vi "CAN MESSAGE.vi"(0 "interface":refnum<k21>, 1 "CAN frame":T1 {"payload" format="%x"; "timestamp" format="%<%.7X\n%x>T"; "type" items=["CAN Data"=0, "CAN Remote"=1, "CAN Bus Error"=2, "CAN 2.0 Data"=8, "CAN FD Data"=16, "CAN FD+BRS Data"=24, "J1939 Data"=192, "Delay"=224, "Log Trigger"=225, "Start Trigger"=226]; "identifier" format="%x"}) -> (2 "cluster":T3 {"data[0]"."payload" format="%x"; "data[0]"."timestamp" format="%<%.7X\n%x>T"; "data[0]"."type" items=["CAN Data"=0, "CAN Remote"=1, "CAN Bus Error"=2, "CAN 2.0 Data"=8, "CAN FD Data"=16, "CAN FD+BRS Data"=24, "J1939 Data"=192, "Delay"=224, "Log Trigger"=225, "Start Trigger"=226]; "data[0]"."identifier" format="%x"; "data[1]"."payload" format="%x"; "data[1]"."timestamp" format="%<%.7X\n%x>T"; "data[1]"."type" items=["CAN Data"=0, "CAN Remote"=1, "CAN Bus Error"=2, "CAN 2.0 Data"=8, "CAN FD Data"=16, "CAN FD+BRS Data"=24, "J1939 Data"=192, "Delay"=224, "Log Trigger"=225, "Start Trigger"=226]; "data[1]"."identifier" format="%x"; "data[2]"."payload" format="%x"; "data[2]"."timestamp" format="%<%.7X\n%x>T"; "data[2]"."type" items=["CAN Data"=0, "CAN Remote"=1, "CAN Bus Error"=2, "CAN 2.0 Data"=8, "CAN FD Data"=16, "CAN FD+BRS Data"=24, "J1939 Data"=192, "Delay"=224, "Log Trigger"=225, "Start Trigger"=226]; "data[2]"."identifier" format="%x"; "data[3]"."payload" format="%x"; "data[3]"."timestamp" format="%<%.7X\n%x>T"; "data[3]"."type" items=["CAN Data"=0, "CAN Remote"=1, "CAN Bus Error"=2, "CAN 2.0 Data"=8, "CAN FD Data"=16, "CAN FD+BRS Data"=24, "J1939 Data"=192, "Delay"=224, "Log Trigger"=225, "Start Trigger"=226]; "data[3]"."identifier" format="%x"; "data[4]"."payload" format="%x"; "data[4]"."timestamp" format="%<%.7X\n%x>T"; "data[4]"."type" items=["CAN Data"=0, "CAN Remote"=1, "CAN Bus Error"=2, "CAN 2.0 Data"=8, "CAN FD Data"=16, "CAN FD+BRS Data"=24, "J1939 Data"=192, "Delay"=224, "Log Trigger"=225, "Start Trigger"=226]; "data[4]"."identifier" format="%x"; "data[5]"."payload" format="%x"; "data[5]"."timestamp" format="%<%.7X\n%x>T"; "data[5]"."type" items=["CAN Data"=0, "CAN Remote"=1, "CAN Bus Error"=2, "CAN 2.0 Data"=8, "CAN FD Data"=16, "CAN FD+BRS Data"=24, "J1939 Data"=192, "Delay"=224, "Log Trigger"=225, "Start Trigger"=226]; "data[5]"."identifier" format="%x"; "data[6]"."payload" format="%x"; "data[6]"."timestamp" format="%<%.7X\n%x>T"; "data[6]"."type" items=["CAN Data"=0, "CAN Remote"=1, "CAN Bus Error"=2, "CAN 2.0 Data"=8, "CAN FD Data"=16, "CAN FD+BRS Data"=24, "J1939 Data"=192, "Delay"=224, "Log Trigger"=225, "Start Trigger"=226]; "data[6]"."identifier" format="%x"; "data[7]"."payload" format="%x"; "data[7]"."timestamp" format="%<%.7X\n%x>T"; "data[7]"."type" items=["CAN Data"=0, "CAN Remote"=1, "CAN Bus Error"=2, "CAN 2.0 Data"=8, "CAN FD Data"=16, "CAN FD+BRS Data"=24, "J1939 Data"=192, "Delay"=224, "Log Trigger"=225, "Start Trigger"=226]; "data[7]"."identifier" format="%x"; "data[8]"."payload" format="%x"; "data[8]"."timestamp" format="%<%.7X\n%x>T"; "data[8]"."type" items=["CAN Data"=0, "CAN Remote"=1, "CAN Bus Error"=2, "CAN 2.0 Data"=8, "CAN FD Data"=16, "CAN FD+BRS Data"=24, "J1939 Data"=192, "Delay"=224, "Log Trigger"=225, "Start Trigger"=226]; "data[8]"."identifier" format="%x"}, 4 "error out":errorcluster)   [LabVIEW 2022 SP3]
uses:
  <vilib>/xnet/xnet.llb/XNET Frame CAN.ctl
  <vilib>/xnet/xnet.llb/XNET Frame Type CAN.ctl
  <vilib>/xnet/xnet.llb/XNET Create Session (Frame Input Stream).vi
  <vilib>/xnet/xnet.llb/XNET Create Session (Frame Output Queued).vi
  <vilib>/xnet/xnet.llb/XNET Write (Frame CAN).vi
  <vilib>/xnet/xnet.llb/XNET Read (Frame CAN).vi
  <resource>/objmgr/xnet.rc
panel:
  in  "error in (no error) 2":errorcluster
  in  "error in (no error)":errorcluster
  in  "DATA IN":T1[](array[typedef]) {"payload" format="%x"; "timestamp" format="%<%.7X\n%x>T"; "type" items=["CAN Data"=0, "CAN Remote"=1, "CAN Bus Error"=2, "CAN 2.0 Data"=8, "CAN FD Data"=16, "CAN FD+BRS Data"=24, "J1939 Data"=192, "Delay"=224, "Log Trigger"=225, "Start Trigger"=226]; "identifier" format="%x"}
  out "data 2":T1[](array[typedef]) {"payload" format="%x"; "timestamp" format="%<%.7X\n%x>T"; "type" items=["CAN Data"=0, "CAN Remote"=1, "CAN Bus Error"=2, "CAN 2.0 Data"=8, "CAN FD Data"=16, "CAN FD+BRS Data"=24, "J1939 Data"=192, "Delay"=224, "Log Trigger"=225, "Start Trigger"=226]; "identifier" format="%x"}
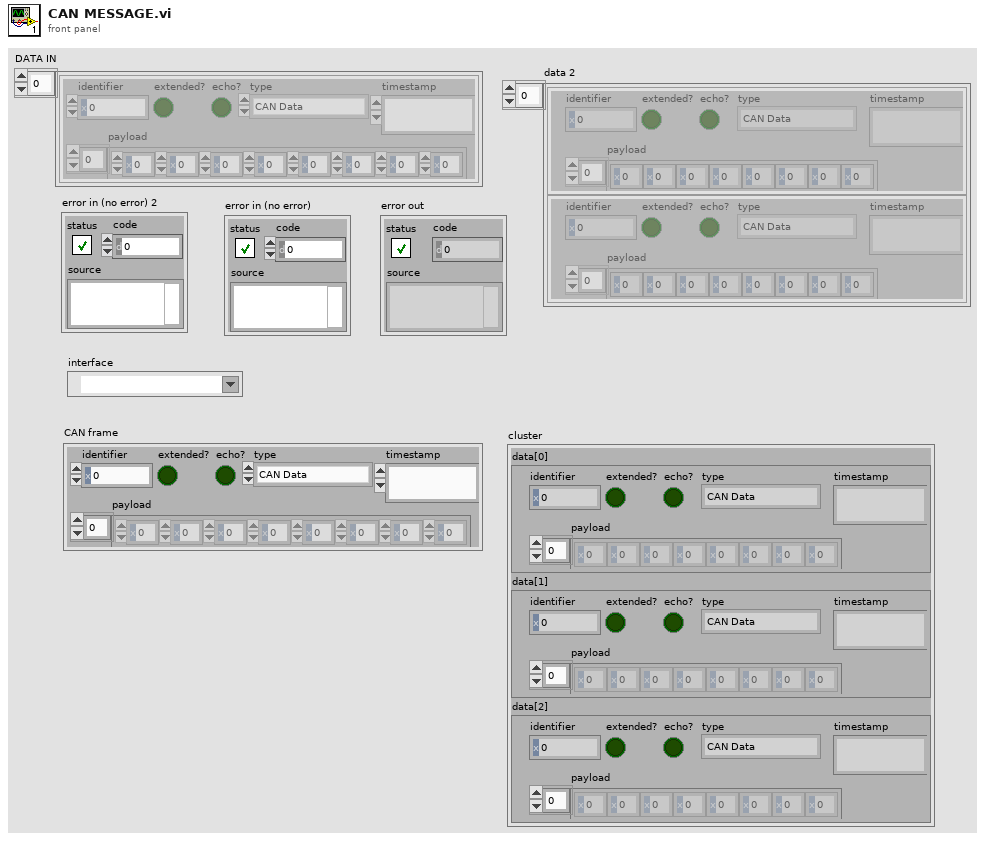
[diagram p1: front panel]
types:
  T1 = typedef "XNET Frame CAN.ctl" = cluster{"timestamp":timestamp, "payload":u8[], "identifier":u32, "type":T2, "extended?":bool, "echo?":bool}
  T2 = typedef "XNET Frame Type CAN.ctl" = u8
  T3 = cluster{"data[0]":T1, "data[1]":T1, "data[2]":T1, "data[3]":T1, "data[4]":T1, "data[5]":T1, "data[6]":T1, "data[7]":T1, "data[8]":T1}
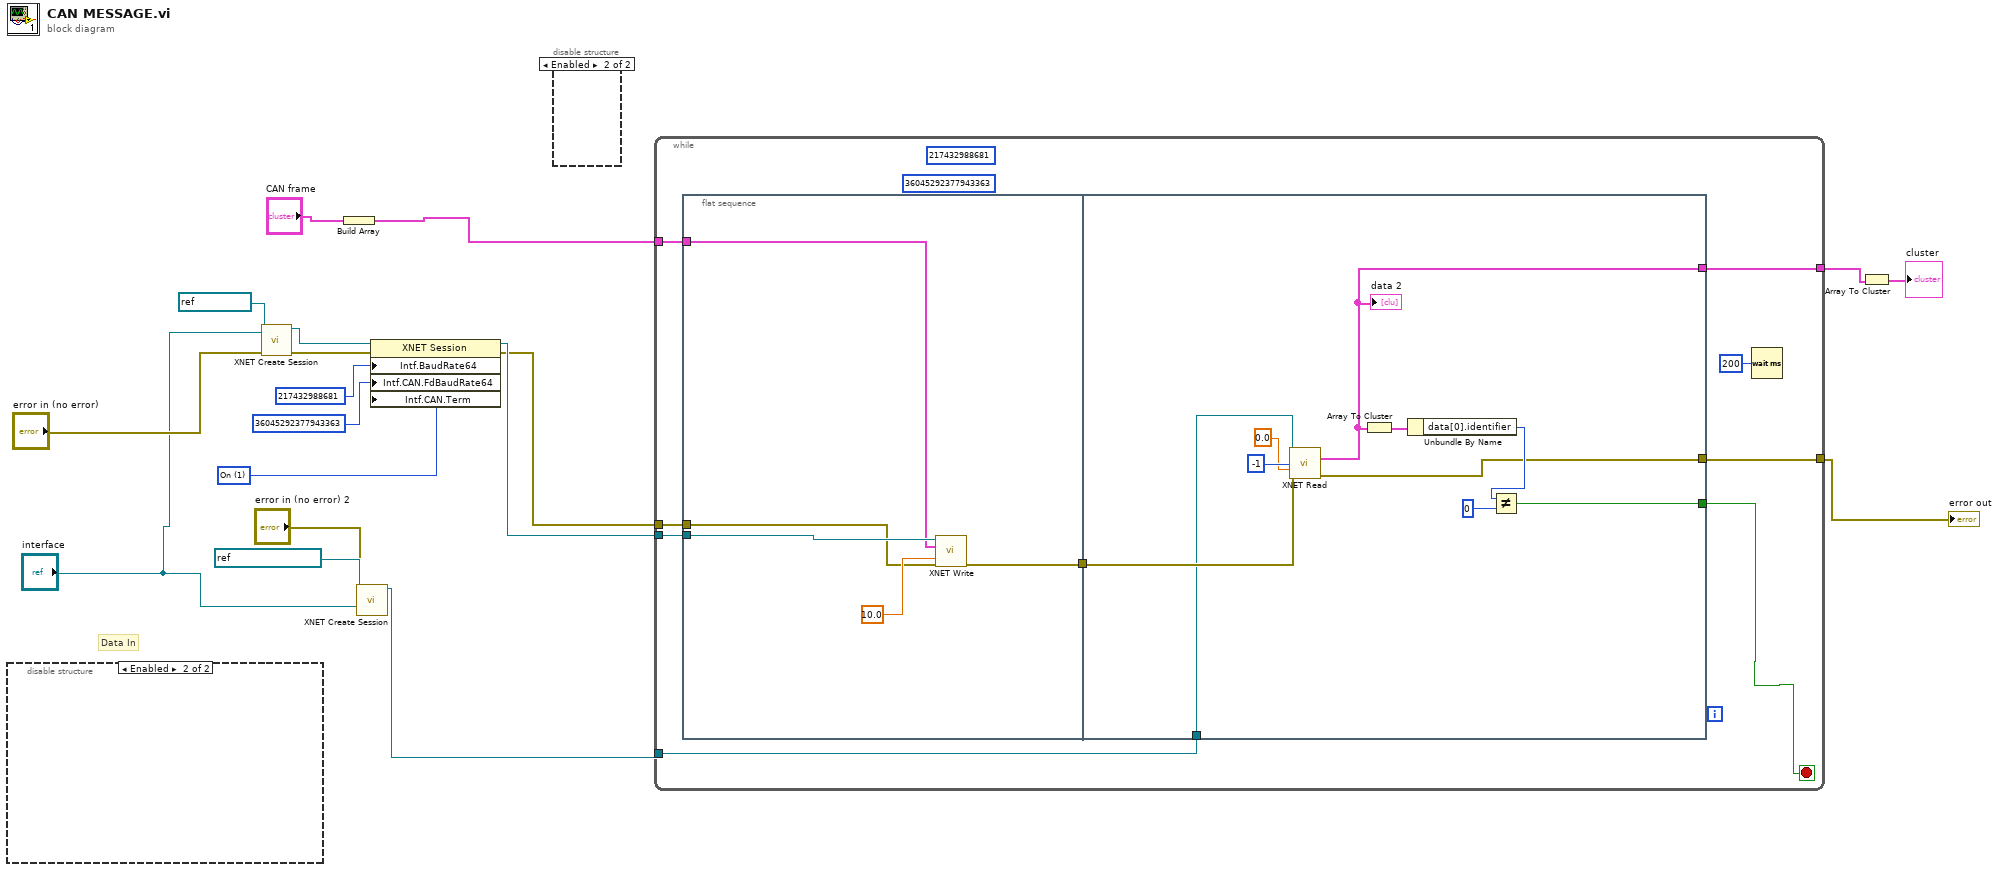
[diagram p0: block diagram]
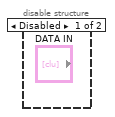
[diagram p2: hidden frame]
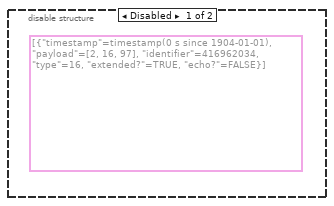
[diagram p3: hidden frame]
diagram:
  w10 = u32 1 items=["Off", "On"] ("Interface:CAN:Termination")
  # "Data In"
  n1 = disable-structure shown="Enabled" {
    frame Disabled {
      (unwired) T1[] [{"timestamp"=timestamp(0 s since 1904-01-01), "payload"=[2, 16, 97], "identifier"=416962034, "type"=16, "extended?"=TRUE, "echo?"=FALSE}] ("data")
    }
    frame Enabled {
    }
  }
  n2 = call-poly <vilib>:"XNET Create Session.vi"("frame"=refnum<k21> "Escritura\nElatch_Labview", "interface"="interface", "error in (no error)"="error in (no error)") -> ("session out"=w5:refnum<k21>, "error out"=w18:errorcluster)  [unwired: 11 in]
  n3 = Build Array("CAN frame") -> (w2:T1[])
  n4 = call-poly <vilib>:"XNET Create Session.vi"("cluster (:memory:)"=refnum<k21> "Elatch_Labview", "interface"="interface", "error in (no error)"="error in (no error) 2") -> ("session out"=w15:refnum<k21>)  [unwired: 11 in, 1 out]
  n5 = property class="XNET Session"(reference=w5, error in=w18, "Intf.BaudRate64"=u64 217432988681 ("Interface:64bit Baud Rate"), "Intf.CAN.FdBaudRate64"=u64 36045292377943363 ("Interface:CAN:64bit FD Baud Rate"), "Intf.CAN.Term"=w10) -> (reference out=w12:refnum<k21>, error out=w11:errorcluster)
  n6 = disable-structure shown="Enabled" {
    frame Disabled {
    }
    frame Enabled {
    }
  }
  n7 = while {
    tunnel: w15 -> [w24]
    tunnel: w12 -> [w27]
    tunnel: w11 -> [w26]
    tunnel: [w22] -> w1
    tunnel: [w21] -> w7
    tunnel: w2 -> [w20]
    stop <- w19 stop-if-true
    (unwired) u64 36045292377943363 ("Interface:CAN:64bit FD Baud Rate")
    (unwired) u64 217432988681 ("Interface:64bit Baud Rate")
    n8 = flat-sequence {
      tunnel: w27 -> [w32]
      tunnel: w26 -> [w30]
      tunnel: [w29] -> w25
      tunnel: w20 -> [w28]
      tunnel: [w38] -> w19
      tunnel: w25 -> [w37]
      tunnel: w24 -> [w36]
      tunnel: [w35] -> w22
      tunnel: [w34] -> w21
      frame #0 {
        n9 = call-poly <vilib>:"XNET Write.vi"("session in"=w32, "data"=w28, "timeout (10)"=10.0, "error in (no error)"=w30) -> ("error out"=w29:errorcluster)  [unwired: 10 in, 1 out]
      }
      frame #1 {
        n10 = call-poly <vilib>:"XNET Read.vi"("session in"=w36, "number to read (-1)"=-1, "timeout (0)"=0.0, "error in (no error)"=w37) -> ("data"=w34:T1[], "error out"=w35:errorcluster)  [unwired: 8 in, 2 out]
        "data 2" <- w34
        n11 = Array To Cluster(array=w34) -> (cluster=w33:T3)
        n12 = Unbundle By Name(w33) -> ("data[0].identifier"=w39:u32)
        n13 = Not Equal?(x=w39, y=u32 0) -> (x != y?=w38:bool)
      }
    }
    n14 = Wait (ms)(milliseconds to wait=u32 200) -> ()  [unwired: 1 out]
  }
  "error out" <- w1
  n15 = Array To Cluster(array=w7) -> (cluster=→"cluster":T3)
